vi "run_autoMemtest_noise.vi"(4 "ExpPhase":string, 6 "control label":string, 8 "error in":errorcluster, 9 "data in":T1={"daq_ao 1"="Dev1/ao0", "daq_ai 1"="Dev1/ai0", "experiment day folder"=path "D:/DATA/8-27-15 save func testing/test.lvm", "Multiclamp init error"=0, "Multiclamp Handle Out"=0, "sampling rate (Hz)"=10000, "trial name"=""}, 10 "clamp switch (T=v, F=i)":bool, 11 "controls array":refnum<vi>[](array[refnum])) -> (0 "error out":errorcluster, 1 "data out":T1={"daq_ao 1"="Dev1/ao0", "daq_ai 1"="Dev1/ai0", "experiment day folder"=path "D:/DATA/8-27-15 save func testing/test.lvm", "Multiclamp init error"=0, "Multiclamp Handle Out"=0, "sampling rate (Hz)"=10000, "trial name"=""}, 2 "cell quality bad":bool, 3 "controls out":refnum<vi>[](array[refnum]), 5 "cell stats":T2 {"STD" format="%010.2f"; "Variance" format="%010.2f"; "Rt (MOhms)" format="%010.2f"; "tau (ms)" format="%08.2g"; "Cm (pF)" format="%08.2f"; "Ra (MOhms)" format="%010.2f"; "Rm (MOhms)" format="%010.2f"; "Ihold (pA)" format="%010.2f"})   [LabVIEW 2019]
uses:
  wc_protocol_v1.003 Folder/whole_cell_protocol/Controls/cell_stats-v02.ctl
  wc_protocol_v1.003 Folder/whole_cell_protocol/Controls/metadata_to_save.ctl
  get_data_from_control_memtest.vi
  Controls/Data.ctl
panel:
  out "Recorded signal (mV or pA)":waveform(dbl)[](graph)
  out "view memtest":waveform(dbl)[](graph)
  # "AUTO RUN WC MEMTEST"
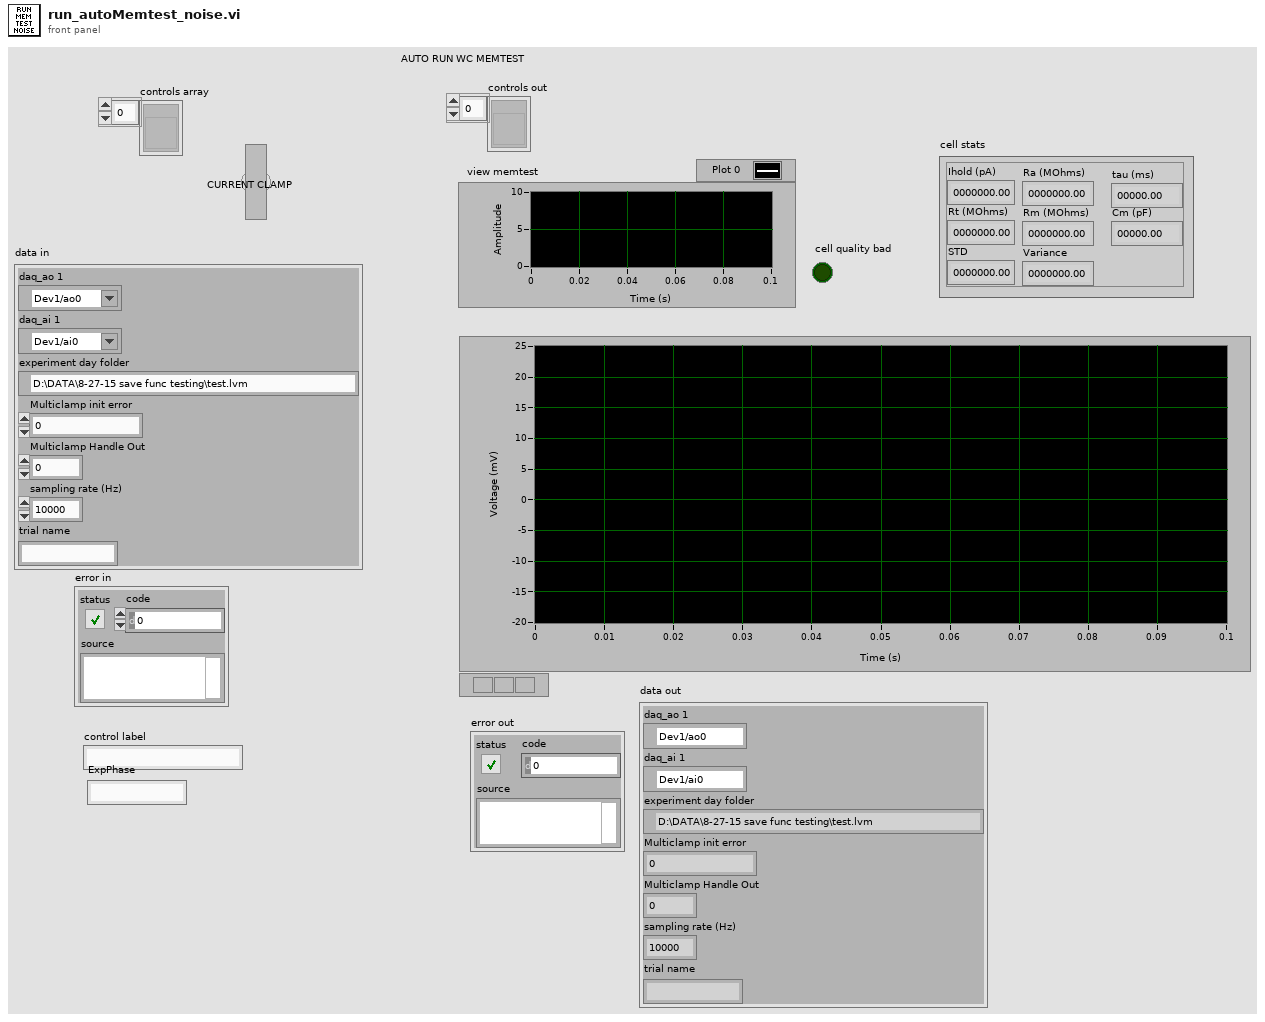
[diagram p1: front panel]
types:
  T1 = typedef "Data.ctl" = cluster{"daq_ao 1":tag, "daq_ai 1":tag, "experiment day folder":path, "Multiclamp init error":i32, "Multiclamp Handle Out":u32, "sampling rate (Hz)":i32, "trial name":string}
  T2 = typedef "cell_stats-v02.ctl" = cluster{"Ihold (pA)":dbl, "Rm (MOhms)":dbl, "Ra (MOhms)":dbl, "Cm (pF)":dbl, "tau (ms)":dbl, "Rt (MOhms)":dbl, "Variance":dbl, "STD":dbl}
  T3 = typedef "memtest_def.ctl" = cluster{"Samples to Read":i32, "Rate (Hz)":dbl, "Amplitude (mV/pA)":dbl, "Offset (mV/pA)":dbl, "Frequency (Hz)":dbl, "duty cycle (%)":dbl, "phase":dbl}
  T4 = typedef "metadata_to_save.ctl" = cluster{"cell stats":T2}
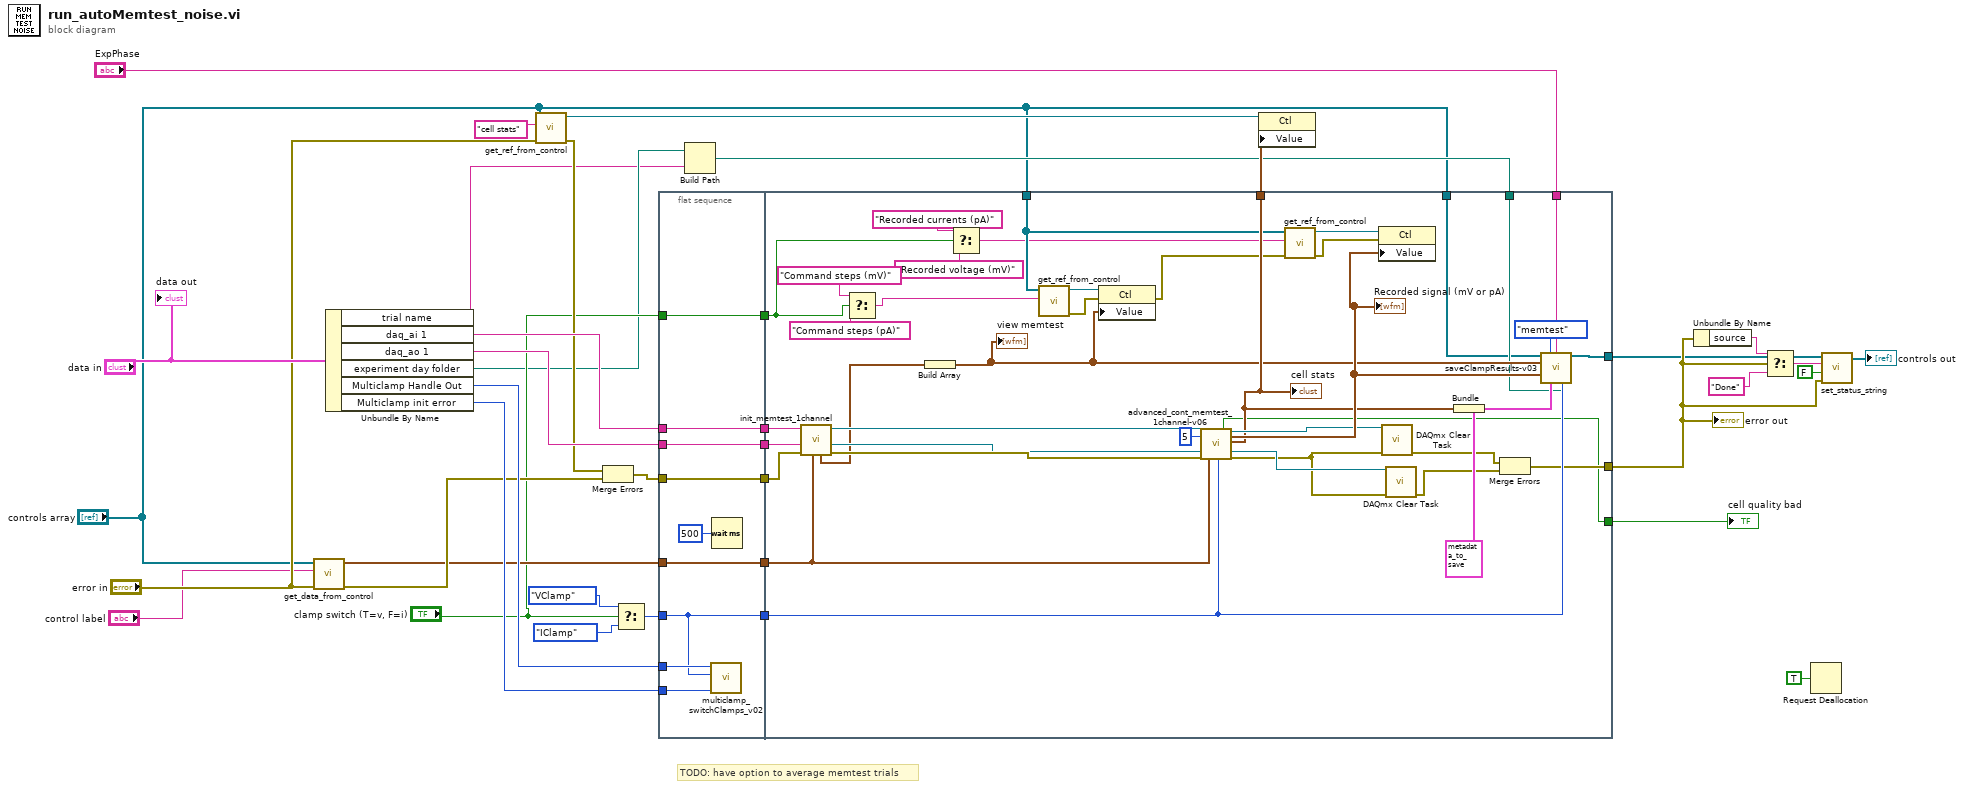
[diagram p0: block diagram]
diagram:
  # "TODO: have option to average memtest trials"
  n1 = call-poly "get_data_from_control.vi"("error in"="error in", "control label"="control label", "controls array"="controls array") -> ("error out"=w14:errorcluster, "memtest output"=w13:T3)  [unwired: 7 in]
  n2 = Unbundle By Name("data in") -> ("trial name"=w7:string, "daq_ai 1"=w30:tag, "daq_ao 1"=w29:tag, "experiment day folder"=w9:path, "Multiclamp Handle Out"=w28:u32, "Multiclamp init error"=w27:i32)
  n3 = call "get_ref_from_control.vi"("error in"="error in", "control label"="cell stats", "controls array"="controls array") -> ("error out"=w20:errorcluster, "reference out"=w25:refnum<vi>)  [unwired: 7 in]
  n4 = Merge Errors(w20, w14) -> (w22:errorcluster)
  n5 = Select(t=enum16{"VClamp", "IClamp"}."VClamp" ("which clamp"), s="clamp switch (T=v, F=i)", f=enum16{"VClamp", "IClamp"}."IClamp" ("which clamp")) -> (s? t:f=w36:enum16{"VClamp", "IClamp"})
  n6 = flat-sequence {
    tunnel: w36 -> [w43]
    tunnel: w30 -> [w47]
    tunnel: [w47] -> w35
    tunnel: w29 -> [w46]
    tunnel: [w46] -> w34
    tunnel: w28 -> [w45]
    tunnel: w27 -> [w44]
    tunnel: [w43] -> w33
    tunnel: [w41] -> w32
    tunnel: w13 -> [w41]
    tunnel: w22 -> [w40]
    tunnel: [w40] -> w21
    tunnel: "clamp switch (T=v, F=i)" -> [w39]
    tunnel: [w39] -> w10
    tunnel: w35 -> [w81]
    tunnel: w34 -> [w80]
    tunnel: w33 -> [w75]
    tunnel: w32 -> [w79]
    tunnel: w8 -> [w55]
    tunnel: [w74] -> w24
    tunnel: w21 -> [w73]
    tunnel: [w70] -> w15
    tunnel: "controls array" -> [w63]
    tunnel: w10 -> [w59]
    tunnel: "controls array" -> [w54]
    tunnel: [w53] -> w5
    tunnel: "ExpPhase" -> [w52]
    tunnel: [w48] -> w2
    frame #0 {
      n7 = call "multiclamp_switchClamps_v02.vi"("error in"=w44, "which clamp"=w43, "Multiclamp Handle in"=w45) -> ()  [unwired: 7 in, 2 out]
      n8 = Wait (ms)(milliseconds to wait=u32 500) -> ()  [unwired: 1 out]
    }
    frame #1 {
      n9 = call "init_memtest_1channel.vi"("memtest"=w79, "AO error in"=w73, "AO physical channels"=w80, "AI Physical Channels"=w81) -> ("AO error out"=w84:errorcluster, "AO task out"=w83:refnum<k21>, "AI task out"=w82:refnum<k21>, "view memtest"=w49:waveform(dbl))  [unwired: 3 in, 1 out]
      n10 = Select(t="Command steps (mV)", s=w59, f="Command steps (pA)") -> (s? t:f=w67:string)
      n11 = Build Array(w49) -> (w69:waveform(dbl)[])
      "view memtest" <- w69
      n12 = Select(t="Recorded currents (pA)", s=w59, f="Recorded voltage (mV)") -> (s? t:f=w58:string)
      n13 = call "get_ref_from_control.vi"("control label"=w67, "controls array"=w63) -> ("error out"=w64:errorcluster, "reference out"=w68:refnum<vi>)  [unwired: 8 in]
      n14 = property class="Ctl"(reference=w68, error in=w64, "Value"=w69) -> (error out=w56:errorcluster)  [unwired: 1 out]
      n15 = call "advanced_cont_memtest_1channel-v06.vi"("Pulse AI task in"=w82, "replicates"=5, "Pulse AO task in"=w83, "error in"=w84, "memtest"=w79, "which clamp"=w75) -> ("cell quality bad"=w48:bool, "Pulse AI task out"=w85:refnum<k21>, "data out (pA or mV)"=w87:waveform(dbl)[], "cell stats"=w74:T2, "Pulse AO task out"=w86:refnum<k21>, "error out"=w50:errorcluster)  [unwired: 5 in, 3 out]
      "cell stats" <- w74
      "Recorded signal (mV or pA)" <- w87
      n16 = call "get_ref_from_control.vi"("error in"=w56, "control label"=w58, "controls array"=w63) -> ("error out"=w57:errorcluster, "reference out"=w62:refnum<vi>)  [unwired: 7 in]
      n17 = property class="Ctl"(reference=w62, error in=w57, "Value"=w87) -> ()  [unwired: 2 out]
      n18 = call <vilib>:"DAQmx Clear Task.vi"("task in"=w85, "error in"=w50) -> ("error out"=w72:errorcluster)  [unwired: 13 in]
      n19 = call <vilib>:"DAQmx Clear Task.vi"("task in"=w86, "error in"=w50) -> ("error out"=w71:errorcluster)  [unwired: 13 in]
      n20 = Bundle(cluster=T4 {"cell stats"={"Ihold (pA)"=0.0, "Rm (MOhms)"=0.0, "Ra (MOhms)"=0.0, "Cm (pF)"=0.0, "tau (ms)"=0.0, "Rt (MOhms)"=0.0, "Variance"=0.0, "STD"=0.0}} ("metadata to save"), "cell stats"=w74) -> (w78:T4)
      n21 = Merge Errors(w72, w71) -> (w70:errorcluster)
      n22 = call "saveClampResults-v03.vi"("controls array"=w54, "protocol or memtest"=enum16{"protocol", "memtest"}."memtest", "ExpPhase"=w52, "which clamp"=w75, "view profile"=w69, "rec profile"=w87, "metadata to save"=w78, "Save to (folder dir)"=w55) -> ("controls array out"=w53:refnum<vi>[])  [unwired: 6 in, 1 out]
    }
  }
  n23 = Build Path(base path=w9, name or relative path=w7) -> (appended path=w8:path)
  n24 = property class="Ctl"(reference=w25, "Value"=w24) -> ()  [unwired: 1 in, 2 out]
  n25 = Unbundle By Name(w15) -> ("source"=w17:string)
  n26 = Select(t=w17, s=w15, f="Done") -> (s? t:f=w18:string)
  n27 = Request Deallocation(TRUE ("flag")) -> ()
  n28 = call "set_status_string.vi"("error in"=w15, "new line?"=FALSE, "status string in"=w18, "controls array"=w5) -> ("controls array out"=→"controls out":refnum<vi>[])  [unwired: 6 in, 1 out]
  "error out" <- w15
  "data out" <- "data in"
  "cell quality bad" <- w2
